vi "ReadControls.vi"(6 "Agents class path":path=path "F:/LVSCC/LV2009/GPL/lib.lib/LVOOP/HGF_MobileAgentSystem/MoAgSy_Scripting/TestAgent/TestAgent/TestAgent.lvclass", 10 "error in (no error)":errorcluster, 11 "vi path":path=path "F:/LVSCC/LV2009/GPL/lib.lib/LVOOP/HGF_MobileAgentSystem/MoAgSy_Scripting/TestAgent/TestAgent/PubVI_1.vi") -> (0 "Controls Cluster":T1(array[cluster]), 2 "error out":errorcluster, 3 "dup vi path":path=path "F:/Scripting/PubVI.vi")   [LabVIEW 2009, in "HGF_VisitorGenerator.lvlib"]
doc: "Read public VIs controls and indicators linked to the connector pane"
uses:
  HGF_VisitorGenerator.lvlib
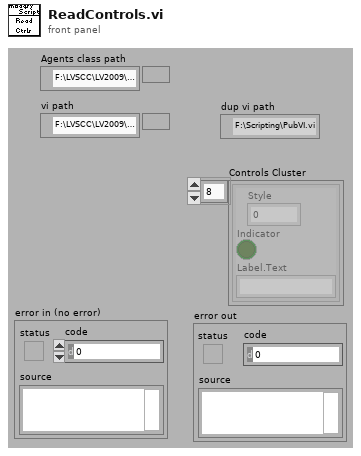
[diagram p1: front panel]
types:
  T1 = cluster{"Style":u32, "Indicator":bool, "Label.Text":string}[]
  T2 = cluster{"Style":u32, "Indicator":bool, "Label.Text":string}
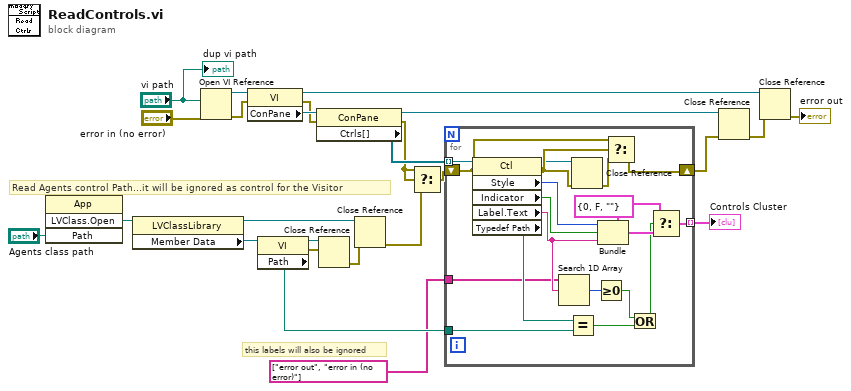
[diagram p0: block diagram]
diagram:
  # "this labels will also be ignored"
  # "Read Agents control Path...it will be ignored as control for the Visitor"
  n1 = invoke class="App" method="LVClass.Open"("Path"="Agents class path") -> ("LVClass.Open"=w11:refnum<vi>)  [unwired: 3 in, 3 out]
  n2 = property class="LVClassLibrary"(reference=w11) -> (reference out=w6:refnum<vi>, "Member Data"=w10:refnum<vi>)  [unwired: 1 in, 1 out]
  n3 = Open VI Reference(vi path="vi path", error in (no error)="error in (no error)") -> (vi reference=w15:refnum<vi>, error out=w13:errorcluster)  [unwired: 4 in]
  n4 = property class="VI"(reference=w15, error in=w13) -> (reference out=w14:refnum<vi>, error out=w20:errorcluster, "ConPane"=w22:refnum<vi>)
  n5 = property class="VI"(reference=w10) -> (reference out=w8:refnum<vi>, error out=w9:errorcluster, "Path"=w2:path)  [unwired: 1 in]
  n6 = property class="ConPane"(reference=w22, error in=w20) -> (reference out=w18:refnum<vi>, error out=w4:errorcluster, "Ctrls[]"=w21:refnum<vi>[])
  n7 = Close Reference(reference=w8, error in (no error)=w9) -> (error out=w7:errorcluster)
  n8 = Close Reference(reference=w6, error in (no error)=w7) -> (error out=w5:errorcluster)
  n9 = Select(t=w4, s=w4, f=w5) -> (s? t:f=w3:errorcluster)
  n10 = for {
    tunnel: w21 -> [w42] mode=indexing
    shift-right: [w37] -> w17
    shift-left: w3 -> [w44]
    tunnel: [w32] -> w19 mode=indexing
    tunnel: w2 -> [w35]
    tunnel: string[] ["error out", "error in (no error)"] -> [w26]
    w36 = T2 {"Style"=0, "Indicator"=FALSE, "Label.Text"=""} ("output cluster")
    n11 = property class="Ctl"(reference=w42, error in=w44) -> (reference out=w39:refnum<vi>, error out=w43:errorcluster, "Style"=w41:u32, "Indicator"=w40:bool, "Label.Text"=w29:string, "Typedef Path"=w31:path)
    n12 = Search 1D Array(1D array=w26, element=w29) -> (index of element=w28:i32)  [unwired: 1 in]
    n13 = Equal?(x=w31, y=w35) -> (x = y?=w34:bool)
    n14 = Close Reference(reference=w39, error in (no error)=w43) -> (error out=w38:errorcluster)
    n15 = Greater Or Equal To 0?(x=w28) -> (x >= 0?=w27:bool)
    n16 = Bundle(cluster=w36, "Style"=w41, "Indicator"=w40, "Label.Text"=w29) -> (w33:T2)
    n17 = Select(t=w44, s=w43, f=w38) -> (s? t:f=w37:errorcluster)
    n18 = Or(x=w27, y=w34) -> (x .or. y?=w30:bool)
    n19 = Select(t=w36, s=w30, f=w33) -> (s? t:f=w32:T2)
  }
  "Controls Cluster" <- w19
  n20 = Close Reference(reference=w18, error in (no error)=w17) -> (error out=w16:errorcluster)
  n21 = Close Reference(reference=w14, error in (no error)=w16) -> (error out=→"error out":errorcluster)
  "dup vi path" <- "vi path"
